vi "NewPort_PM_Test.vi"(11 "PM Count":i32=1 min=1 max=4 step=1) -> (0 "Error":errorcluster, 3 "CMD Query":string[](array[string]))   [LabVIEW 2017]
uses:
  C:/Program Files (x86)/Newport/Newport USB Driver/Bin/UsbDllWrap.dll
  Program Files (x86)/Newport/Newport USB Driver/Bin/UsbDllWrap.dll
panel:
  out "reference Out":refnum<k24>
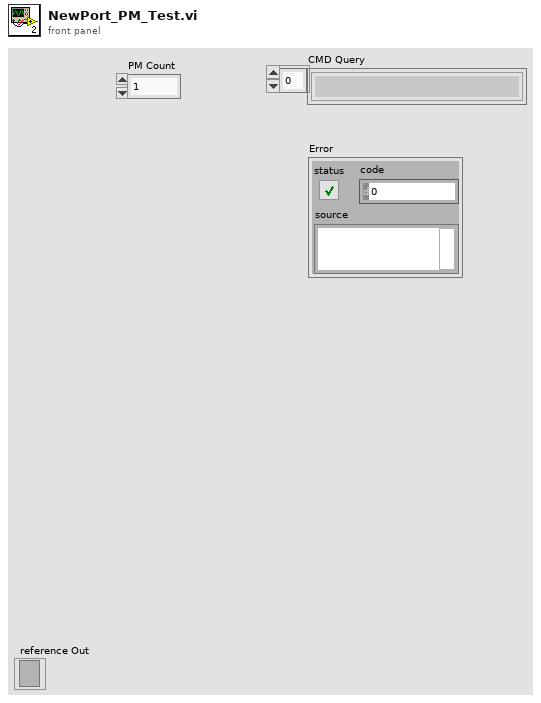
[diagram p1: front panel]
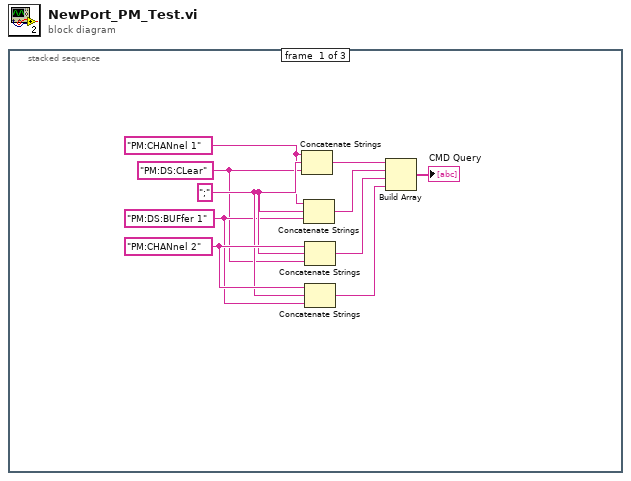
[diagram p0: block diagram]
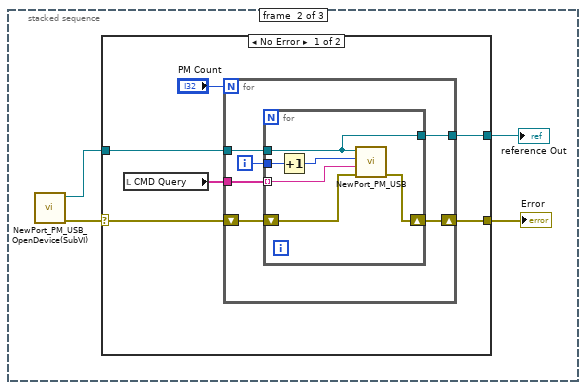
[diagram p2: hidden frame]
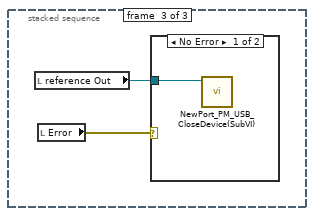
[diagram p4: hidden frame]
diagram:
  n1 = stacked-sequence {
    frame #0 {
      w5 = "PM:CHANnel 2" ("PM:CMD_QUERY In")
      w3 = "PM:DS:BUFfer 1" ("PM:CMD_QUERY In")
      w4 = ";" ("PM:CMD_QUERY In")
      w2 = "PM:DS:CLear" ("PM:CMD_QUERY In")
      w1 = "PM:CHANnel 1" ("PM:CMD_QUERY In")
      n2 = Concatenate Strings(w1, w4, w2) -> (w6:string)
      n3 = Concatenate Strings(w1, w4, w3) -> (w7:string)
      n4 = Concatenate Strings(w5, w4, w2) -> (w8:string)
      n5 = Concatenate Strings(w5, w4, w3) -> (w9:string)
      n6 = Build Array(w6, w7, w8, w9) -> (→"CMD Query":string[])
    }
    frame #1 {
      n7 = call "NewPort_PM_USB_OpenDevice(SubVI).vi"() -> ("error out"=w14:errorcluster, "reference Out"=w13:refnum<k24>)  [unwired: 10 in]
      n8 = case shown="No Error" w14 {
        selector: w14 -> [w19 w34]
        tunnel: w13 -> [w18 w33]
        tunnel: [w16 w34] -> w12
        tunnel: [w15 w33] -> w11
        frame No Error {
          n9 = local read "CMD Query"() -> (w17:string[])
          n10 = for {
            N: "PM Count" -> [_]
            tunnel: w18 -> [w26]
            tunnel: w17 -> [w22]
            shift-right: [w24] -> w16
            shift-left: w19 -> [w25]
            tunnel: [w21] -> w15
            i -> [w23]
            n11 = for {
              tunnel: w26 -> [w27]
              shift-right: [w31] -> w24
              shift-left: w25 -> [w32]
              tunnel: w23 -> [w30]
              tunnel: w22 -> [w28] mode=indexing
              tunnel: [w27] -> w21
              n12 = Increment(x=w30) -> (x+1=w29:i32)
              n13 = call "NewPort_PM_USB.vi"("error in"=w32, "PM:CMD_QUERY In"=w28, "USB Address"=w29, "reference"=w27) -> ("error out"=w31:errorcluster)  [unwired: 5 in, 2 out]
            }
          }
        }
        frame Error {
        }
      }
      "Error" <- w12
      "reference Out" <- w11
    }
    frame #2 {
      n14 = local read "reference Out"() -> (w35:refnum<k24>)
      n15 = local read "Error"() -> (w36:errorcluster)
      n16 = case shown="No Error" w36 {
        tunnel: w35 -> [w37 _]
        frame No Error {
          n17 = call "NewPort_PM_USB_CloseDevice(SubVI).vi"("reference In"=w37) -> ()  [unwired: 10 in, 1 out]
        }
        frame Error {
        }
      }
    }
  }
